vi "Update Generic Counter Value.vi"(8 "Increment?":bool, 11 "Input Counter Val":u16) -> (3 "Updated Counter Val":u16)   [LabVIEW 2012]
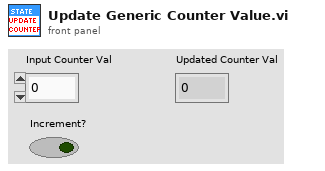
[diagram p1: front panel]
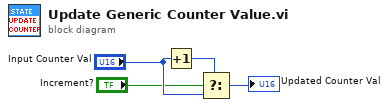
[diagram p0: block diagram]
diagram:
  n1 = Increment(x="Input Counter Val") -> (x+1=w4:u16)
  n2 = Select(t=w4, s="Increment?", f="Input Counter Val") -> (s? t:f=→"Updated Counter Val":u16)
